vi "Errorbar0008.vi"   [LabVIEW 2013]
uses:
  <vilib>/Heliosphere Research LLC/Advanced Plotting Toolkit/api_core/NewPlotScales.ctl
  <vilib>/Heliosphere Research LLC/Advanced Plotting Toolkit/Advanced Plotting Toolkit.lvlib
types:
  T1 = typedef "Advanced Plotting Toolkit.lvlib/NewPlotScales.ctl" = enum16{"Default", "Linear", "Log", "Symlog"}
  T2 = typedef "Advanced Plotting Toolkit.lvlib/PlotID.ctl" = i32
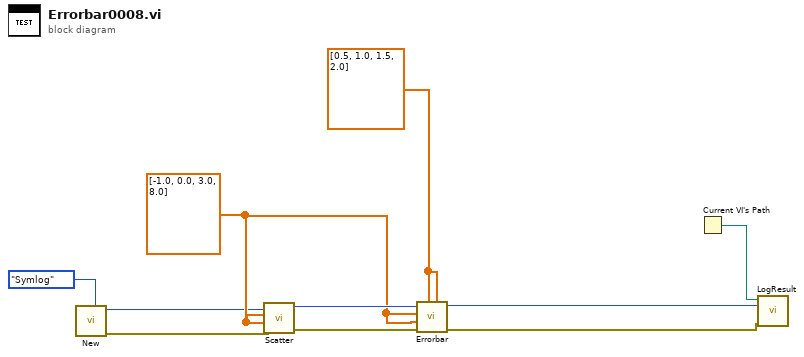
[diagram p0: block diagram]
diagram:
  w4 = dbl[] [0.5, 1.0, 1.5, 2.0] ("X Errors")
  w5 = dbl[] [-1.0, 0.0, 3.0, 8.0] ("X Data")
  n1 = call <vilib>:"New.vi"("Y Axis Scale"=NewPlotScales."Symlog") -> ("error out"=w1:errorcluster, "Plot ID"=w2:T2)  [unwired: 9 in]
  n2 = call <vilib>:"Scatter.vi"("error in (no error)"=w1, "Y Data"=w5, "X Data"=w5, "Plot ID"=w2) -> ("error out"=w6:errorcluster, "Plot ID Out"=w7:T2)  [unwired: 6 in]
  n3 = call <vilib>:"Errorbar.vi"("Y Errors"=w4, "X Errors"=w4, "error in (no error)"=w6, "Y Data"=w5, "X Data"=w5, "Plot ID"=w7) -> ("error out"=w8:errorcluster, "Plot ID out"=w9:T2)  [unwired: 4 in]
  n4 = Current VI's Path() -> (path=w10:path)
  n5 = call "LogResult.vi"("Test Result"=w8, "Test Artifact"=w9, "VI Path"=w10) -> ()  [unwired: 9 in]
